vi "Dymin_RT_Main.vi"() -> ()   [LabVIEW 2016]
doc: "The myRIO Custom FPGA Project template acquires button data from the onboard button and displays the button value on a Boolean indicator. The SYS.RDY indicator shows the FPGA status."
uses:
  Z:/C/PM100D/Calibrate_control.ctl
  <vilib>/userdefined/High Color/nirio_resource_hc.ctl
  <vilib>/myRIO/Common/Instrument Driver Framework/myRIO v1.0/UART/vis/myRIO v1.0 Close UART.vi
  <vilib>/FPGAPlugInAG/myRIO-1900/niLvFpga_Open_myRIO-1900.vi
  <vilib>/rvi/interface/common/dynamic/niFpgaDynamicAddResources.vi
  <vilib>/Utility/error.llb/Error Cluster From Error Code.vi
  <vilib>/rvi/errors/niLvFpgaAdjustHostInterfaceError.vi
  <vilib>/FPGAPlugInAG/Dynamic/niLvFpga_Close_Dynamic.vi
  <vilib>/myRIO/Common/Instrument Driver Framework/Utilities/vis/FPGA Ref Manager.vi
  <vilib>/myRIO/Common/Instrument Driver Framework/myRIO v1.0/myRIO v1.0 Reset FPGA.vi
  <vilib>/myRIO/Common/Instrument Driver Framework/myRIO v1.0/IRQ/vis/myRIO v1.0 IRQ Info FGV.vi
  <vilib>/myRIO/Common/Instrument Driver Framework/myRIO v1.0/IRQ/vis/myRIO v1.0 Timer IRQ Info FGV.vi
  <vilib>/myRIO/Common/Instrument Driver Framework/myRIO v1.0/IRQ/vis/myRIO v1.0 ISR Agent.vi
  <vilib>/rvi/interface/nirviOpenFPGA/nirviOpenFPGA.xnode
  FPGA Bitfiles/Dymin4ALL_FPGATarget_DyminFPGAMain2_ryjuvA8w6JM.lvbitx
  Dymin_FPGA_Main.vi
  <vilib>/express/express arith-compare/Formula/XNode/ExpressFormulaBlockNode.xnode
  <vilib>/rvi/interface/nirviReadWriteControl/nirviReadWriteControl.xnode
  <vilib>/rvi/interface/nirviCloseFPGA/nirviCloseFPGA.xnode
  <vilib>/myRIO/Instrument Drivers/Utilities/Utilities.lvlib
  NiFpgaLv.dll
  <vilib>/rvi/interface/Simulation/niFpgaSimulationCallBeginRW.vi
panel:
  in  "AOM Power":dbl[](array[numeric])=[0.0, 0.0, 0.0, 0.0] min=0.0 max=1.0
  in  "Calibrate?":T1
  in  "error in":errorcluster
  out "All Step Times (us)":dbl[](array[numeric]) min=0.0 max=1.0
  out "PIX CLK period (us)":dbl
  out "PIX CLK period (bits)":i32
  out "PIX CLK Measured (us)":dbl
  in  "DyMIN Step Time (us)":dbl[](array[numeric])=[0.0, 0.0, 0.0, 0.0] min=0.0 max=10000.0 step=0.0125
  in  "Laser Wait (us)":dbl min=0.0 max=100000.0 step=0.0125
  out "PIX CLK Measured (bits)":i32
  in  "Dymin On?":bool
  out "Time (#80MHz periods)":i32[](array[numeric])
  in  "Threshold (counts)":i32[](array[numeric])=[0, 0, 0, 0]
  out "AOM Voltage":dbl[](array[numeric]) min=0.0 max=1.0
  out "error out":errorcluster
  in  "Stop":bool
  # "AOM Voltages:\nIN0=A/AO0\nIN1=C/AO1\nIN2=C/AO0\nIN3=A/AO0\n\nVoltage conversion (raw voltages from FPGA):\nMSP Connectors:\nVoltage=RawDataValue*4.883 mV\nMXP Connectors:\nVoltage=RawDataValue*1.221 mV\nMeasured with 50Ohm\nVoltage=RawDataValue*2.1mV\n\nI have calibrated the program to the voltage output into 50 Ohms, you will need to calibrate it to your system."
  # "Calibrate_enum.ctl\nRequirements: \nLabview 2016 (32 bit)\nLabview Real-Time Module\nLabview FPGA Module\nCompile Cloud access (Sign up at https://www.ni.com/en-us/support/documentation/supplemental/14/compile-faster-with-the-labview-fpga-compile-cloud-service.html)\nOR Xilinx Compilation Tools to compile the code on your FPGA.\n.\nInstructions:\n1. Check the myRIO target IP address in the project and make sure the target IP address is correct. \n2. Run this VI."
  # "SET YOUR PIXEL CLOCK TO THIS VALUE"
  # "Size of time bits\n1 bit=12.5 ns"
  # "Steps including dummy steps"
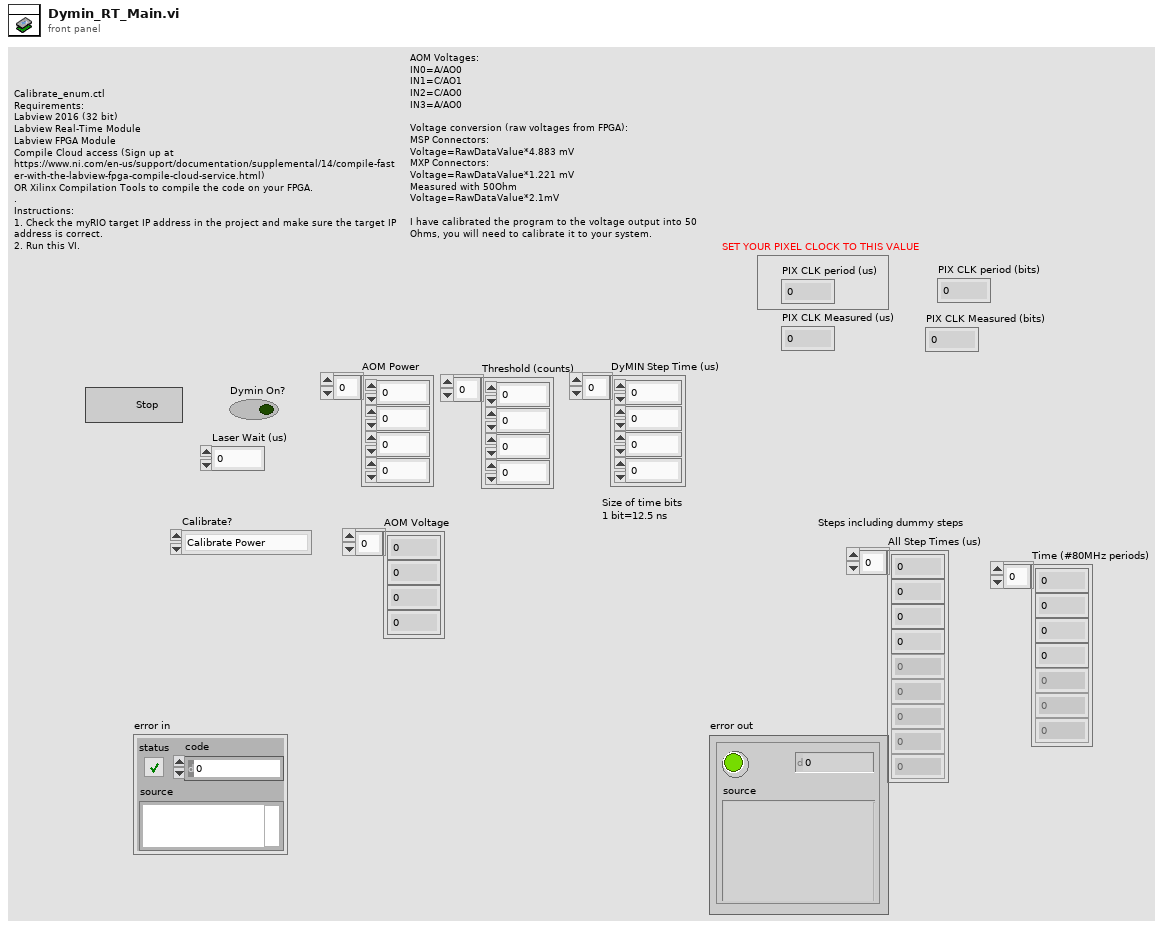
[diagram p1: front panel]
types:
  T1 = typedef "Calibrate_control.ctl" = enum16{"Calibrate Power", "Recall Calibration"}
  T2 = typedef "nirio_resource_hc.ctl" = tag
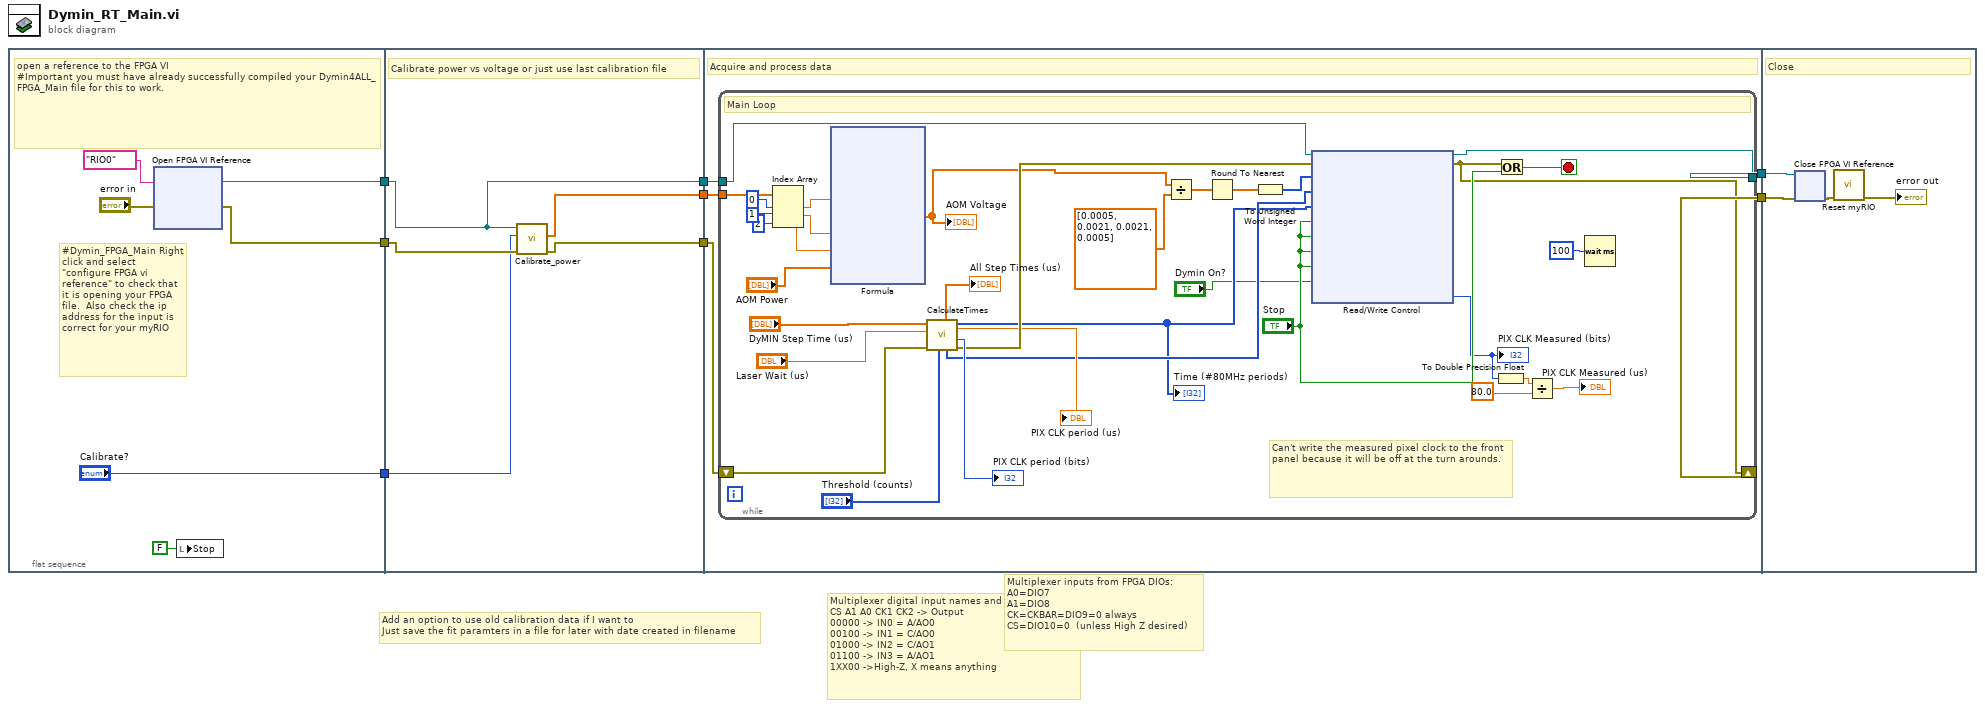
[diagram p0: block diagram]
diagram:
  # "Add an option to use old calibration data if I want to\nJust save the fit paramters in a file for later with date created in filename"
  # "Multiplexer inputs from FPGA DIOs:\nA0=DIO7\nA1=DIO8\nCK=CKBAR=DIO9=0 always\nCS=DIO10=0  (unless High Z desired)"
  # "Multiplexer digital input names and truth table:\nCS A1 A0 CK1 CK2 -> Output\n00000 -> IN0 = A/AO0\n00100 -> IN1 = C/AO0\n01000 -> IN2 = C/AO1\n01100 -> IN3 = A/AO1\n1XX00 ->High-Z, X means anything"
  n1 = flat-sequence {
    tunnel: [w13] -> w6
    tunnel: [w10] -> w5
    tunnel: ["Calibrate?"] -> w4
    tunnel: w6 -> [w17]
    tunnel: w5 -> [w19]
    tunnel: w4 -> [w16]
    tunnel: [w17] -> w3
    tunnel: [w18] -> w2
    tunnel: [w15] -> w1
    tunnel: [w24] -> w8
    tunnel: [w23] -> w7
    tunnel: w3 -> [w22]
    tunnel: w2 -> [w21]
    tunnel: w1 -> [w20]
    tunnel: w8 -> [w81]
    tunnel: w7 -> [w80]
    frame #0 {
      # "#Dymin_FPGA_Main Right click and select \"configure FPGA vi reference\" to check that it is opening your FPGA file.  Also check the ip address for the input is correct for your myRIO"
      # "open a reference to the FPGA VI\n#Important you must have already successfully compiled your Dymin4ALL_FPGA_Main file for this to work."
      n2 = xnode "Open FPGA VI Reference"("error in"="error in", "resource name"=T2 "RIO0") -> ("FPGA VI Reference Out"=w13:refnum<k20>, "error out"=w10:errorcluster)
      n3 = local write "Stop"(FALSE ("Stop")) -> ()
    }
    frame #1 {
      # "Calibrate power vs voltage or just use last calibration file"
      n4 = call "Calibrate_power.vi"("error in"=w19, "Calibrate?"=w16, "FPGA VI Reference IN"=w17) -> ("error out"=w18:errorcluster, "Fit Parameters"=w15:dbl[])  [unwired: 5 in, 2 out]
    }
    frame #2 {
      # "Acquire and process data"
      n5 = while {
        tunnel: w22 -> [w57]
        tunnel: [w55] -> w24
        shift-right: [w42] -> w23
        shift-left: w21 -> [w45]
        tunnel: w20 -> [w25]
        stop <- w58 stop-if-true
        # "Can't write the measured pixel clock to the front panel because it will be off at the turn arounds."
        # "Main Loop"
        n6 = Index Array(array=w25, index #1=0 ("index"), index #2=1 ("index"), index #3=2 ("index")) -> (element #1=w30:dbl, element #2=w29:dbl, element #3=w28:dbl)
        n7 = xnode "Formula"("X1"=w30, "X2"=w29, "X3"=w28, "P"="AOM Power") -> ("Result"=w26:dbl[])  [unwired: 1 in, 1 out]
        "AOM Voltage" <- w26
        n8 = call "CalculateTimes.vi"("Threshold (counts)"="Threshold (counts)", "error in"=w45, "Laser Wait time (us)"="Laser Wait (us)", "DyMIN Step Times (us)"="DyMIN Step Time (us)") -> ("error out"=w40:errorcluster, "PIX CLK period (bits)"=→"PIX CLK period (bits)":i32, "PIX CLK period (us)"=→"PIX CLK period (us)":dbl, "All Step Times (bits)"=w35:i32[], "All Thresholds (counts)"=w36:i32[], "All Step Times (us)"=→"All Step Times (us)":dbl[])  [unwired: 2 in]
        "Time (#80MHz periods)" <- w35
        n9 = Divide(x=w26, y=dbl[] [0.0005, 0.0021, 0.0021, 0.0005]) -> (x/y=w52:dbl[])
        n10 = Round To Nearest(number=w52) -> (nearest integer value=w51:dbl[])
        n11 = To Unsigned Word Integer(number=w51) -> (unsigned 16bit integer=w50:u16[])
        n12 = xnode "Read/Write Control"("FPGA VI Reference In"=w57, "error in"=w40, "AOM Volts"=w50, "Threshold (counts)"=w36, "Time (#80MHz periods)"=w35, "stop 1"="Stop", "stop 2"="Stop", "stop 3"="Stop", "stop 4"="Stop", "Dymin On?"="Dymin On?") -> ("FPGA VI Reference Out"=w55:refnum<k20>, "error out"=w42:errorcluster, "PIX CLK (bits)"=w43:i32)
        "PIX CLK Measured (bits)" <- w43
        n13 = To Double Precision Float(number=w43) -> (double precision float=w48:dbl)
        n14 = Or(x=w42, y="Stop") -> (x .or. y?=w58:bool)
        n15 = Divide(x=w48, y=80.0) -> (x/y=→"PIX CLK Measured (us)":dbl)
        n16 = Wait (ms)(milliseconds to wait=u32 100) -> ()  [unwired: 1 out]
      }
    }
    frame #3 {
      # "Close"
      n17 = xnode "Close FPGA VI Reference"("FPGA VI Reference In"=w81, "error in"=w80) -> ("error out"=w79:errorcluster)
      n18 = call <vilib>:"Reset myRIO.vi"("error in (no error)"=w79) -> ("error out"=→"error out":errorcluster)  [unwired: 10 in]
    }
  }
